vi "setNumberOfSavedImages.vi"(8 "error in (no error)":errorcluster, 10 "NumberOfSavedImages":dbl, 11 "AndorIKonAcquisitor.lvclass in":refnum<class "AndorIKonAcquisitor.lvclass">) -> (0 "error out":errorcluster, 3 "AndorIKonAcquisitor.lvclass out":refnum<class "AndorIKonAcquisitor.lvclass">)   [LabVIEW 2009, in "Hardware.lvlib" / "Channels.lvlib" / "AndorIKonAcquisitor.lvclass"]
uses:
  AndorIKonAcquisitor.lvclass
  AndorIKonAcquisitor.lvclass/AndorIKonAcquisitor.ctl
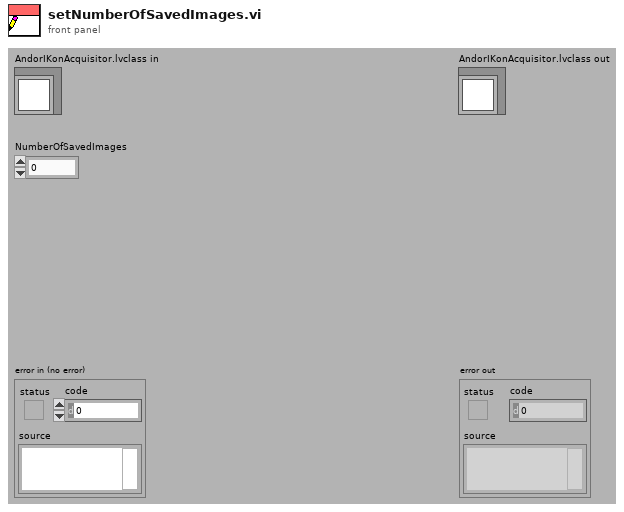
[diagram p1: front panel]
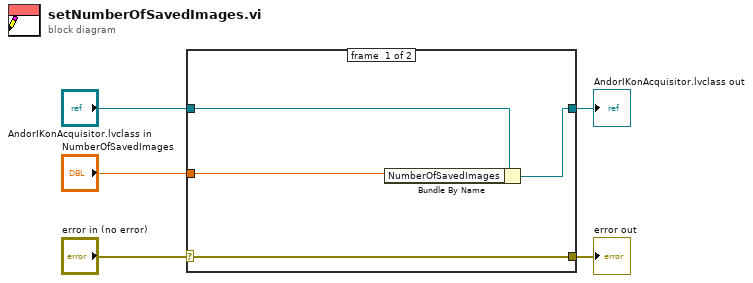
[diagram p0: block diagram]
diagram:
  n1 = case shown="No Error" "error in (no error)" {
    selector: "error in (no error)" -> [w9 w10]
    tunnel: [w9 w10] -> w4
    tunnel: [w7 w11] -> w2
    tunnel: "AndorIKonAcquisitor.lvclass in" -> [w8 w11]
    tunnel: "NumberOfSavedImages" -> [w6 _]
    frame #0 {
      n2 = Bundle By Name(cluster=w8, "NumberOfSavedImages"=w6) -> (w7:refnum<class "AndorIKonAcquisitor.lvclass">)
    }
    frame #1 {
    }
  }
  "error out" <- w4
  "AndorIKonAcquisitor.lvclass out" <- w2
